vi "GetStage.vi"(8 "error in (no error)":errorcluster, 10 "MG17Motor":refnum<k7>, 11 "Microscope in":refnum<class "Microscope.lvclass">) -> (0 "error out":errorcluster, 3 "Microscope out":refnum<class "Microscope.lvclass">)   [LabVIEW 2012, in "Microscope.lvclass"]
uses:
  classes/Microscope.lvclass
  classes/Microscope.lvclass/Microscope.ctl
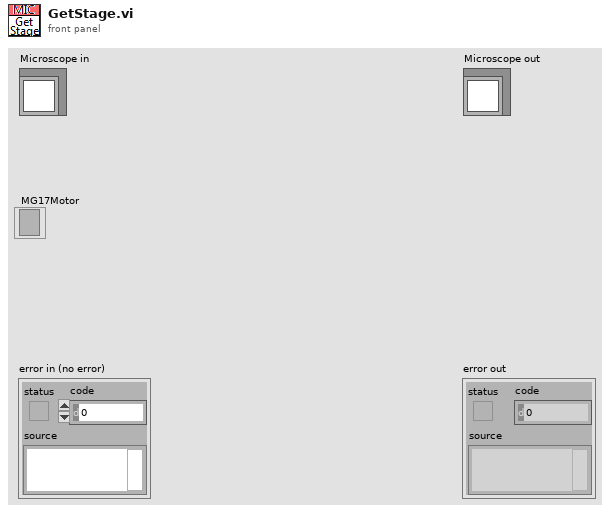
[diagram p1: front panel]
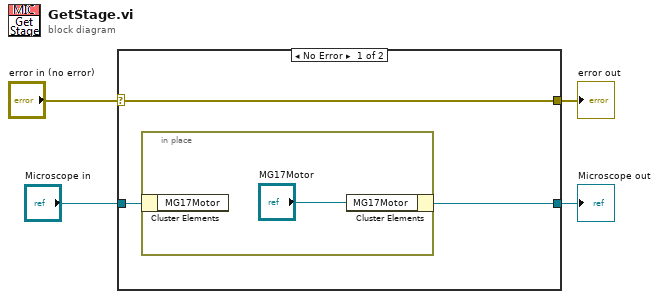
[diagram p0: block diagram]
diagram:
  n1 = case shown="No Error" "error in (no error)" {
    selector: "error in (no error)" -> [w7 w10]
    tunnel: [w7 w10] -> w3
    tunnel: [w5 w9] -> w1
    tunnel: "Microscope in" -> [w6 w9]
    frame No Error {
      n2 = in-place {
        n3 = in-place-cluster #1(w6) -> ()  [unwired: 1 out]
        n4 = in-place-cluster #1("MG17Motor"="MG17Motor") -> (w5:refnum<class "Microscope.lvclass">)
      }
    }
    frame Error {
    }
  }
  "error out" <- w3
  "Microscope out" <- w1
